vi "Update Indicators.vi"(8 "error in (no error)":errorcluster, 11 "Bioreactor in":refnum<class "Bioreactor.lvclass">) -> (0 "error out":errorcluster, 3 "Bioreactor out":refnum<class "Bioreactor.lvclass">)   [LabVIEW 2012, in "Bioreactor Actor.lvlib" / "Bioreactor.lvclass"]
uses:
  Bioreactor.lvclass
  Bioreactor.lvclass/Bioreactor.ctl
  Read DVR.vi
  Read Loop Name.vi
  Read TDMS.vi
  Read Graph History.vi
  Read Process Graph.vi
  Read Control Graph.vi
  Read Process Value.vi
  Read Control Value.vi
  Read Process Setpoint.vi
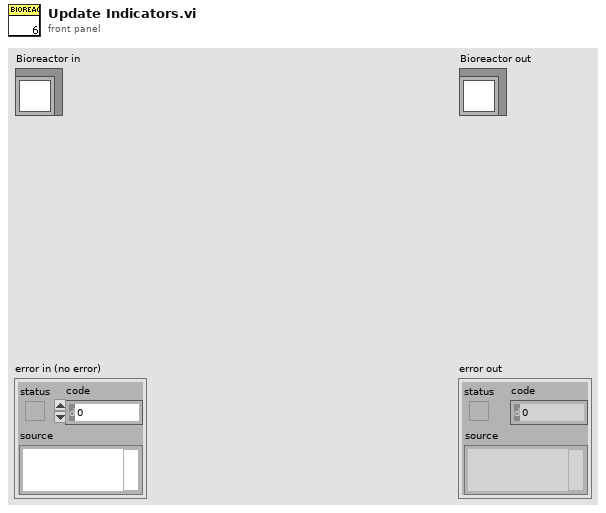
[diagram p1: front panel]
types:
  T1 = cluster{"Name":string, "Value":dbl, "Setpoint":dbl, "Output":dbl}[]
  T2 = cluster{"Name":string, "Value":dbl, "Setpoint":dbl, "Output":dbl}
  T3 = cluster{"output array":dbl[], "output array":dbl[]}
  T4 = cluster{"output array":dbl[], "output array":dbl[]}[]
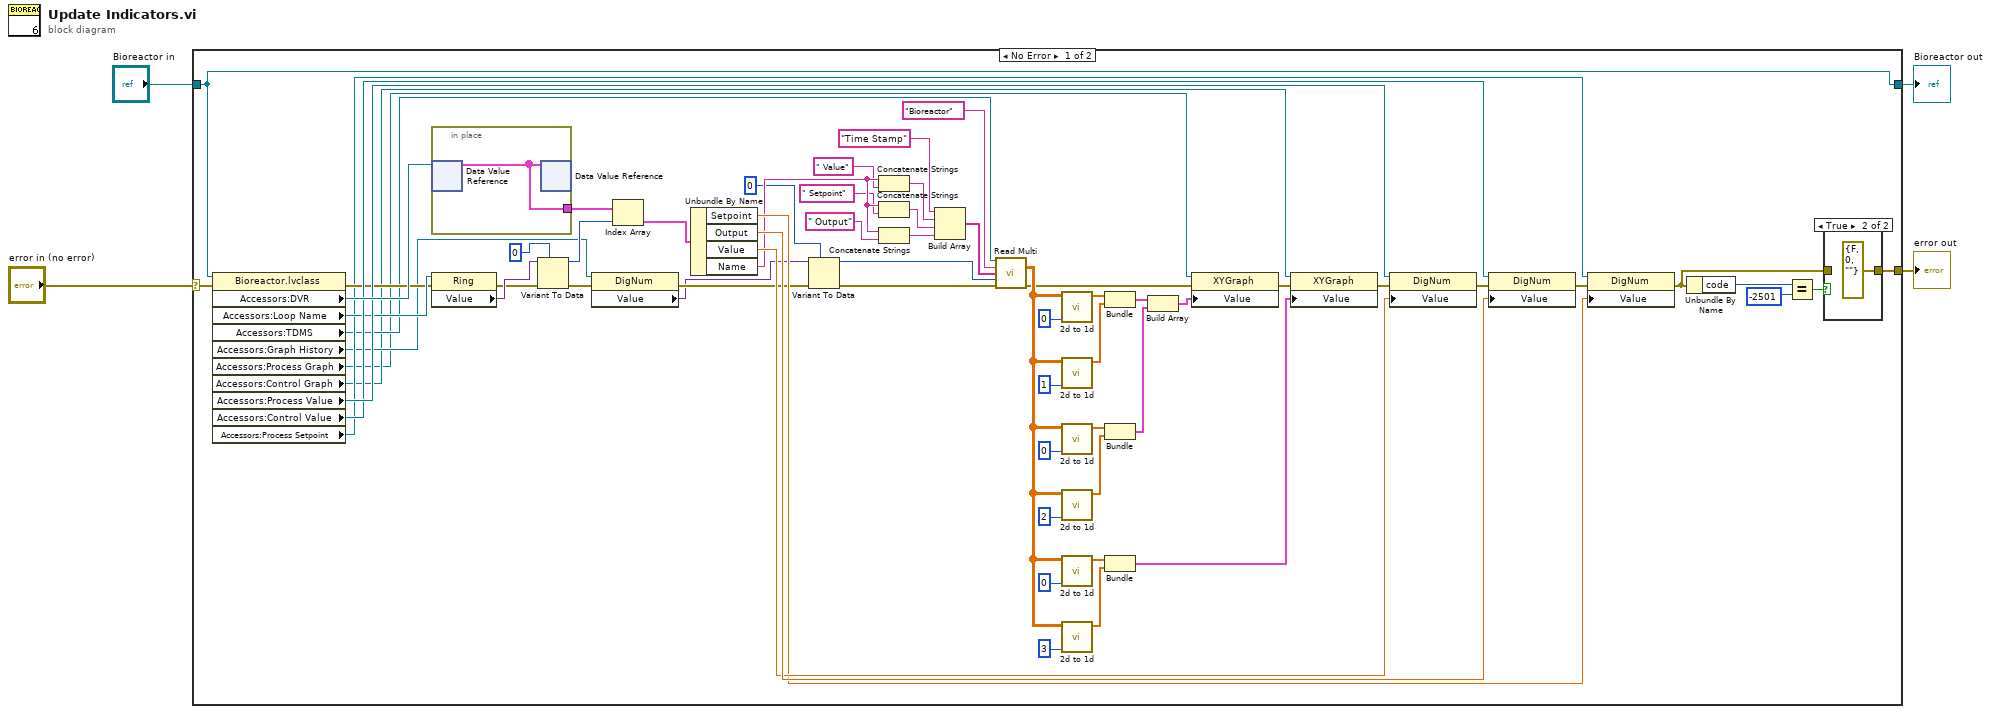
[diagram p0: block diagram]
diagram:
  n1 = case shown="No Error" "error in (no error)" {
    selector: "error in (no error)" -> [w57 w73]
    tunnel: [w5 w73] -> w3
    tunnel: [w68 w72] -> w1
    tunnel: "Bioreactor in" -> [w68 w72]
    frame No Error {
      n2 = property class="Bioreactor.lvclass"(reference=w68, error in=w57) -> (error out=w56:errorcluster, "Accessors:DVR"=w67:refnum<data-value>, "Accessors:Loop Name"=w61:refnum<vi>, "Accessors:TDMS"=w37:refnum<k34>, "Accessors:Graph History"=w26:refnum<vi>, "Accessors:Process Graph"=w24:refnum<vi>, "Accessors:Control Graph"=w25:refnum<vi>, "Accessors:Process Value"=w66:refnum<vi>, "Accessors:Control Value"=w65:refnum<vi>, "Accessors:Process Setpoint"=w50:refnum<vi>)  [unwired: 1 out]
      n3 = in-place {
        in-place-border: [w71] -> w60
        n4 = in-place-dvr #1(w67) -> (w71:T1)  [unwired: 1 out]
        n5 = in-place-dvr #1(w71) -> ()  [unwired: 2 out]
      }
      n6 = property class="Ring"(reference=w61, error in=w56) -> (error out=w62:errorcluster, "Value"=w63:variant)  [unwired: 1 out]
      n7 = Variant To Data(error in=w62, type=0, Variant=w63) -> (data=w59:i32, error out=w21:errorcluster)
      n8 = property class="DigNum"(reference=w26, error in=w21) -> (error out=w41:errorcluster, "Value"=w40:variant)  [unwired: 1 out]
      n9 = Index Array(array=w60, index=w59) -> (element=w58:T2)
      n10 = Unbundle By Name(w58) -> ("Setpoint"=w52:dbl, "Output"=w54:dbl, "Value"=w53:dbl, "Name"=w49:string)
      n11 = Variant To Data(error in=w41, type=0, Variant=w40) -> (data=w38:i32, error out=w22:errorcluster)
      n12 = Concatenate Strings(w49, " Value" ("string")) -> (w45:string)
      n13 = Concatenate Strings(w49, " Setpoint" ("string")) -> (w44:string)
      n14 = Concatenate Strings(w49, " Output" ("string")) -> (w43:string)
      n15 = Build Array("Time Stamp" ("string"), w45, w44, w43) -> (w42:string[])
      n16 = call "Read Multi.vi"("tdms file in"=w37, "group"="Bioreactor", "Channel"=w42, "Numeric"=w38, "error in (no error)"=w22) -> ("Array"=w29:dbl[][], "error out"=w23:errorcluster)  [unwired: 7 in, 2 out]
      n17 = call "2d to 1d.vi"("index"=0, "array"=w29) -> ("output array"=w17:dbl[])  [unwired: 9 in]
      n18 = call "2d to 1d.vi"("index"=1, "array"=w29) -> ("output array"=w16:dbl[])  [unwired: 9 in]
      n19 = call "2d to 1d.vi"("index"=0, "array"=w29) -> ("output array"=w19:dbl[])  [unwired: 9 in]
      n20 = call "2d to 1d.vi"("index"=2, "array"=w29) -> ("output array"=w18:dbl[])  [unwired: 9 in]
      n21 = call "2d to 1d.vi"("index"=0, "array"=w29) -> ("output array"=w12:dbl[])  [unwired: 9 in]
      n22 = call "2d to 1d.vi"("index"=3, "array"=w29) -> ("output array"=w11:dbl[])  [unwired: 9 in]
      n23 = Bundle("output array"=w17, "output array"=w16) -> (w15:T3)  [unwired: 1 in]
      n24 = Bundle("output array"=w19, "output array"=w18) -> (w14:T3)  [unwired: 1 in]
      n25 = Bundle("output array"=w12, "output array"=w11) -> (w10:T3)  [unwired: 1 in]
      n26 = Build Array(w15, w14) -> (w13:T4)
      n27 = property class="XYGraph"(reference=w24, error in=w23, "Value"=w13) -> (error out=w28:errorcluster)  [unwired: 1 out]
      n28 = property class="XYGraph"(reference=w25, error in=w28, "Value"=w10) -> (error out=w27:errorcluster)  [unwired: 1 out]
      n29 = property class="DigNum"(reference=w66, error in=w27, "Value"=w53) -> (error out=w55:errorcluster)  [unwired: 1 out]
      n30 = property class="DigNum"(reference=w65, error in=w55, "Value"=w54) -> (error out=w51:errorcluster)  [unwired: 1 out]
      n31 = property class="DigNum"(reference=w50, error in=w51, "Value"=w52) -> (error out=w6:errorcluster)  [unwired: 1 out]
      n32 = Unbundle By Name(w6) -> ("code"=w9:i32)
      n33 = Equal?(x=w9, y=-2501) -> (x = y?=w7:bool)
      n34 = case shown="True" w7 {
        tunnel: w6 -> [w69 _]
        tunnel: [w69 errorcluster {"status"=FALSE, "code"=0, "source"=""} ("error constant")] -> w5
        frame False {
        }
        frame True {
        }
      }
    }
    frame Error {
    }
  }
  "error out" <- w3
  "Bioreactor out" <- w1
